vi "AOTF signals3 color.vi"() -> ()   [LabVIEW 2020]
uses:
  <vilib>/DAQmx/write.llb/DAQmx Write (Digital 1D Bool 1Chan 1Samp).vi
  <vilib>/DAQmx/write.llb/DAQmx Write (Analog 1D Wfm NChan NSamp).vi
  <vilib>/DAQmx/create/channels.llb/DAQmx Create Channel (AO-Voltage-Basic).vi
  <vilib>/DAQmx/create/channels.llb/DAQmx Create Channel (DO-Digital Output).vi
  <vilib>/DAQmx/configure/timing.llb/DAQmx Timing (Use Waveform).vi
  <vilib>/DAQmx/miscellaneous.llb/DAQmx Fill In Error Info.vi
  <vilib>/measure/NI_MABase.lvlib
panel:
  out "x*y":dbl=32.52032520325203
  out "number of samples written per channel":u32=1
  in  "Stop":bool
  out "LabVIEW generated Sawtooth input (blue) and Camera trigger (red)":waveform(dbl)[](graph)=[{"t0"=timestamp(0 s since 1904-01-01), "dt"=0.001, "Y"=array[3075 elements]}, {"t0"=timestamp(0 s since 1904-01-01), "dt"=0.001, "Y"=array[3075 elements]}, {"t0"=timestamp(0 s since 1904-01-01), "dt"=0.001, "Y"=array[3075 elements]}]
  out "# Samples written per channel 2":u32=3075
  in  "Stop 2":bool
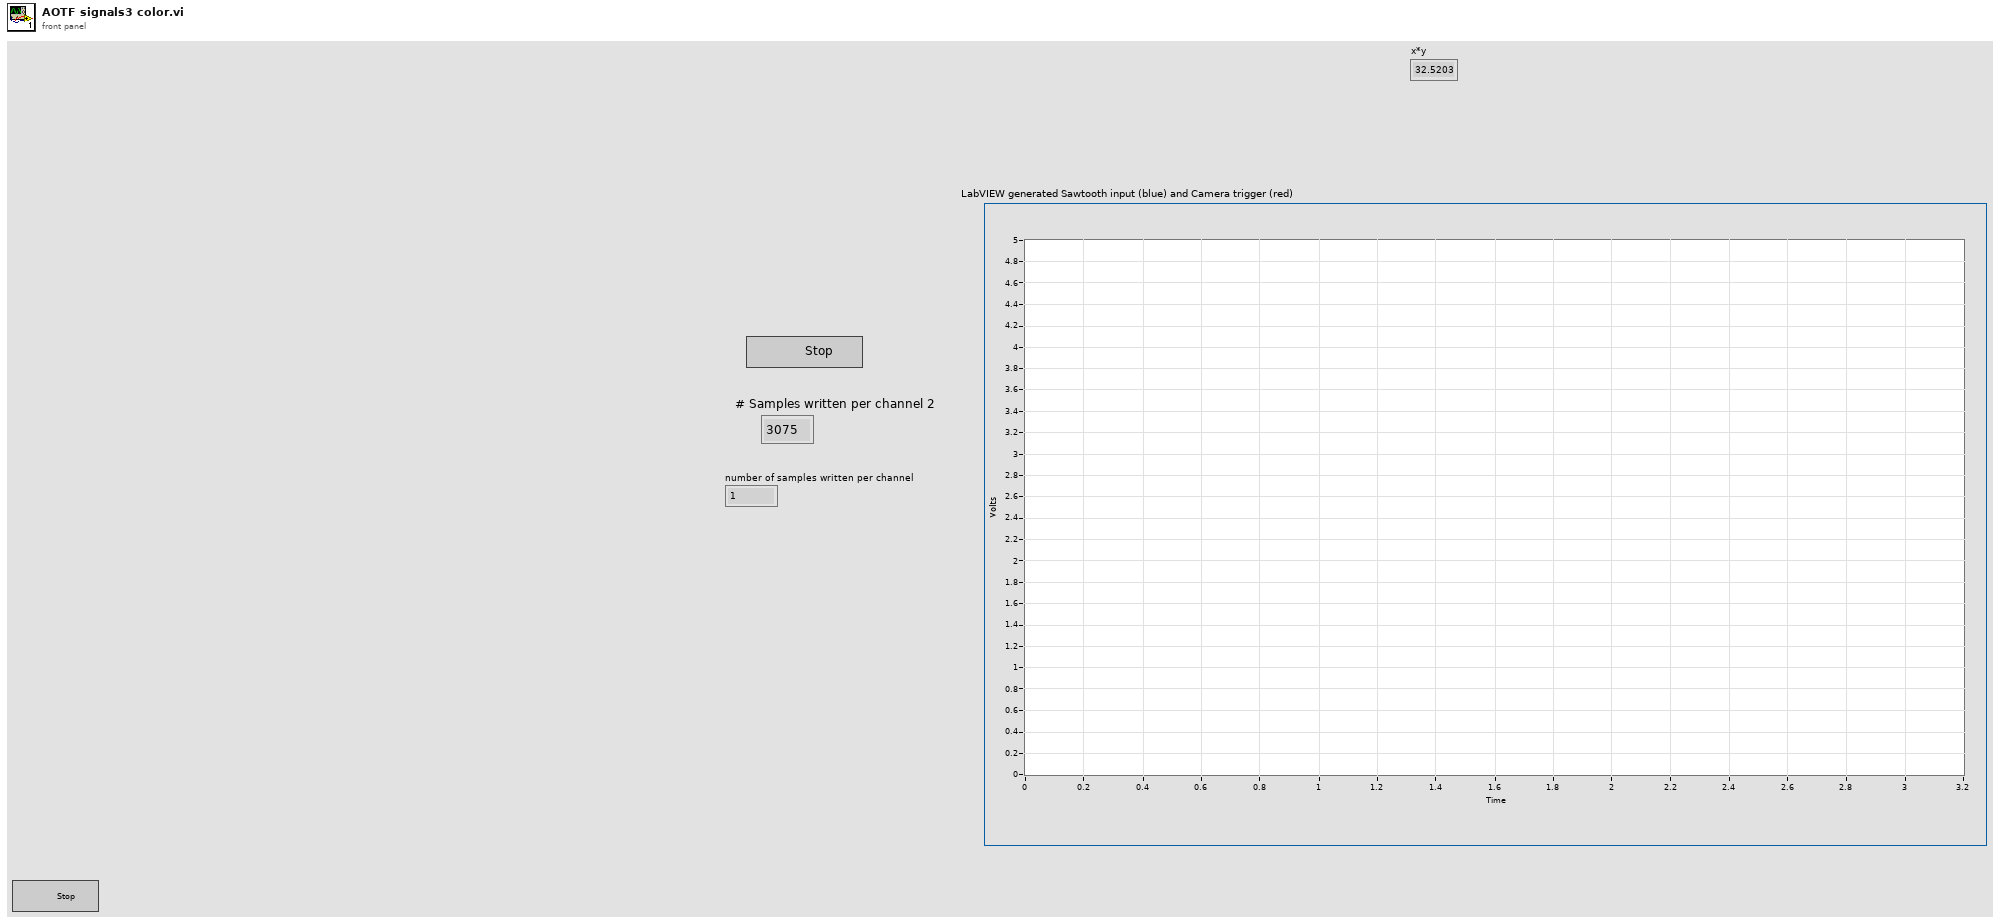
[diagram p1: front panel]
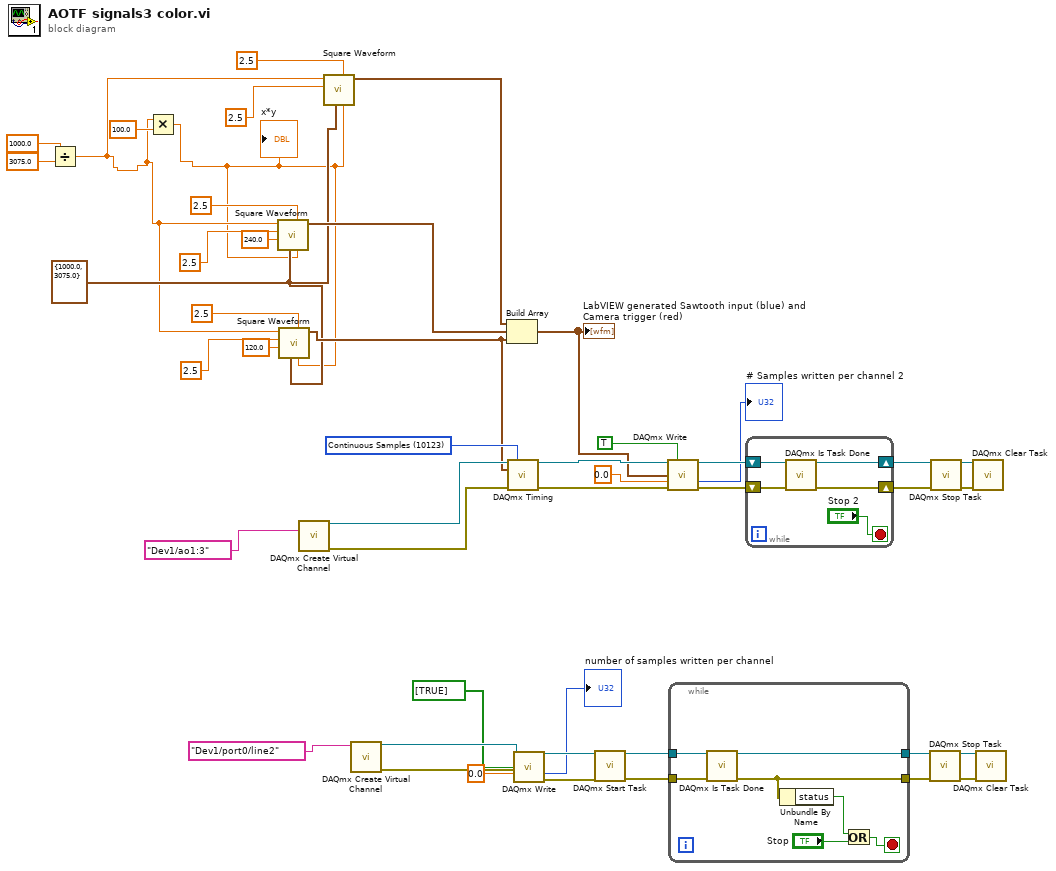
[diagram p0: block diagram]
diagram:
  w7 = cluster{"Fs":dbl, "#s":dbl} {"Fs"=1000.0, "#s"=3075.0} ("sampling info")
  w43 = 10123 items=["Finite Samples"=10178, "Continuous Samples"=10123, "Hardware Timed Single Point"=12522] ("sample mode")
  n1 = Divide(x=1000.0, y=3075.0) -> (x/y=w3:dbl)
  n2 = Multiply(x=w3, y=100.0) -> (x*y=w2:dbl)
  "x*y" <- w2
  n3 = call <vilib>:"Square Waveform.vi"("duty cycle (%)"=w2, "offset"=2.5, "sampling info"=w7, "phase"=240.0, "amplitude"=2.5 ("Amplitude for laser 1 (Max value 2.5)"), "frequency"=w3) -> ("signal out"=w30:waveform(dbl))  [unwired: 4 in, 1 out]
  n4 = call <vilib>:"Square Waveform.vi"("duty cycle (%)"=w2, "offset"=2.5, "sampling info"=w7, "phase"=120.0, "amplitude"=2.5 ("Amplitude for laser 1 (Max value 2.5)"), "frequency"=w3) -> ("signal out"=w27:waveform(dbl))  [unwired: 4 in, 1 out]
  n5 = call-poly <vilib>:"DAQmx Create Virtual Channel.vi"("physical channels"=tag "Dev1/ao1:3") -> ("task out"=w45:refnum<k21>, "error out"=w44:errorcluster)  [unwired: 13 in]
  n6 = call <vilib>:"Square Waveform.vi"("duty cycle (%)"=w2, "offset"=2.5, "sampling info"=w7, "amplitude"=2.5 ("Amplitude for laser 1 (Max value 2.5)"), "frequency"=w3) -> ("signal out"=w5:waveform(dbl))  [unwired: 5 in, 1 out]
  n7 = call-poly <vilib>:"DAQmx Create Virtual Channel.vi"("lines"=tag "Dev1/port0/line2") -> ("task out"=w22:refnum<k21>, "error out"=w21:errorcluster)  [unwired: 13 in]
  n8 = Build Array(w5, w30, w27) -> (w33:waveform(dbl)[])
  "LabVIEW generated Sawtooth input (blue) and Camera trigger (red)" <- w33
  n9 = call-poly <vilib>:"DAQmx Timing.vi"("task/channels in"=w45, "sample mode"=w43, "waveform"=w27, "error in"=w44) -> ("task out"=w40:refnum<k21>, "error out"=w39:errorcluster)  [unwired: 10 in]
  n10 = call-poly <vilib>:"DAQmx Write.vi"("task/channels in"=w22, "data"=bool[] [TRUE], "timeout"=0.0, "error in"=w21) -> ("task out"=w20:refnum<k21>, "number of samples written per channel"=→"number of samples written per channel":u32, "error out"=w19:errorcluster)  [unwired: 9 in]
  n11 = call <vilib>:"DAQmx Start Task.vi"("task/channels in"=w20, "error in"=w19) -> ("task out"=w18:refnum<k21>, "error out"=w17:errorcluster)  [unwired: 12 in]
  n12 = call-poly <vilib>:"DAQmx Write.vi"("task/channels in"=w40, "auto start"=TRUE, "data"=w33, "timeout"=0.0, "error in"=w39) -> ("task out"=w41:refnum<k21>, "number of samples written per channel"=→"# Samples written per channel 2":u32, "error out"=w42:errorcluster)  [unwired: 8 in]
  n13 = while {
    tunnel: w18 -> [w54]
    tunnel: w17 -> [w53]
    tunnel: [w51] -> w13
    tunnel: [w52] -> w14
    stop <- w48 stop-if-true
    n14 = call <vilib>:"DAQmx Is Task Done.vi"("task/channels in"=w54, "error in"=w53) -> ("task out"=w52:refnum<k21>, "error out"=w51:errorcluster)  [unwired: 11 in, 1 out]
    n15 = Unbundle By Name(w51) -> ("status"=w50:bool)
    n16 = Or(x=w50, y="Stop") -> (x .or. y?=w48:bool)
  }
  n17 = while {
    shift-right: [w56] -> w37
    shift-left: w41 -> [w59]
    shift-right: [w57] -> w38
    shift-left: w42 -> [w58]
    stop <- "Stop 2" stop-if-true
    n18 = call <vilib>:"DAQmx Is Task Done.vi"("task/channels in"=w59, "error in"=w58) -> ("task out"=w56:refnum<k21>, "error out"=w57:errorcluster)  [unwired: 11 in, 1 out]
  }
  n19 = call <vilib>:"DAQmx Stop Task.vi"("task/channels in"=w14, "error in"=w13) -> ("task out"=w16:refnum<k21>, "error out"=w15:errorcluster)  [unwired: 12 in]
  n20 = call <vilib>:"DAQmx Stop Task.vi"("task/channels in"=w37, "error in"=w38) -> ("task out"=w46:refnum<k21>, "error out"=w47:errorcluster)  [unwired: 12 in]
  n21 = call <vilib>:"DAQmx Clear Task.vi"("task in"=w46, "error in"=w47) -> ()  [unwired: 13 in, 1 out]
  n22 = call <vilib>:"DAQmx Clear Task.vi"("task in"=w16, "error in"=w15) -> ()  [unwired: 13 in, 1 out]
